vi "Copy Image To Picture.vi"(8 "error in (no error)":errorcluster, 10 "Transparency Threshold (127)":u8=127, 11 "image_ptr":i64) -> (0 "error out":errorcluster, 3 "Picture":T1)   [LabVIEW 2020, in "G-Image.lvlib"]
doc: "Read the image data from the pointer into LabVIEW, then free the memory. The image is returned as a LabVIEW picture."
uses:
  G-Image.lvlib
  <vilib>/picture/picture.llb/imagedata.ctl
  <vilib>/Utility/file.llb/Application Directory.vi
  <vilib>/Utility/error.llb/Error Cluster From Error Code.vi
  lib/g_image_32.dll
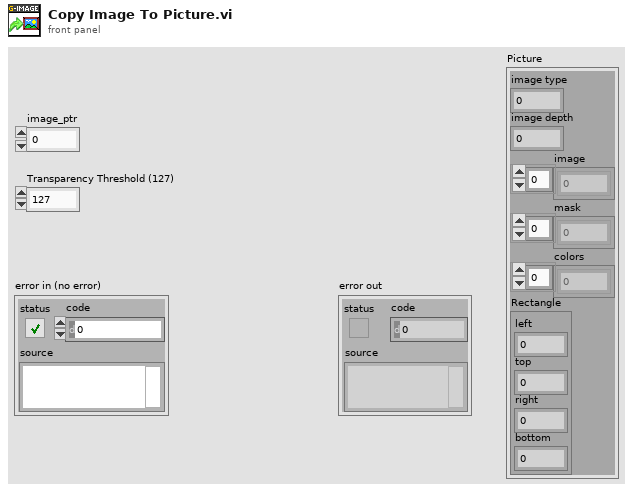
[diagram p1: front panel]
types:
  T1 = typedef "imagedata.ctl" = cluster{"image type":i32, "image depth":i32, "image":u8[], "mask":u8[], "colors":u32[], "Rectangle":cluster{"left":i16, "top":i16, "right":i16, "bottom":i16}}
  T2 = cluster{"data":i32, "colors":i32, "data_size":i32, "color_size":i32, "width":i32, "height":i32, "depth":i32}
  T3 = cluster{"data":i64, "colors":i64, "data_size":i32, "color_size":i32, "width":i32, "height":i32, "depth":i32}
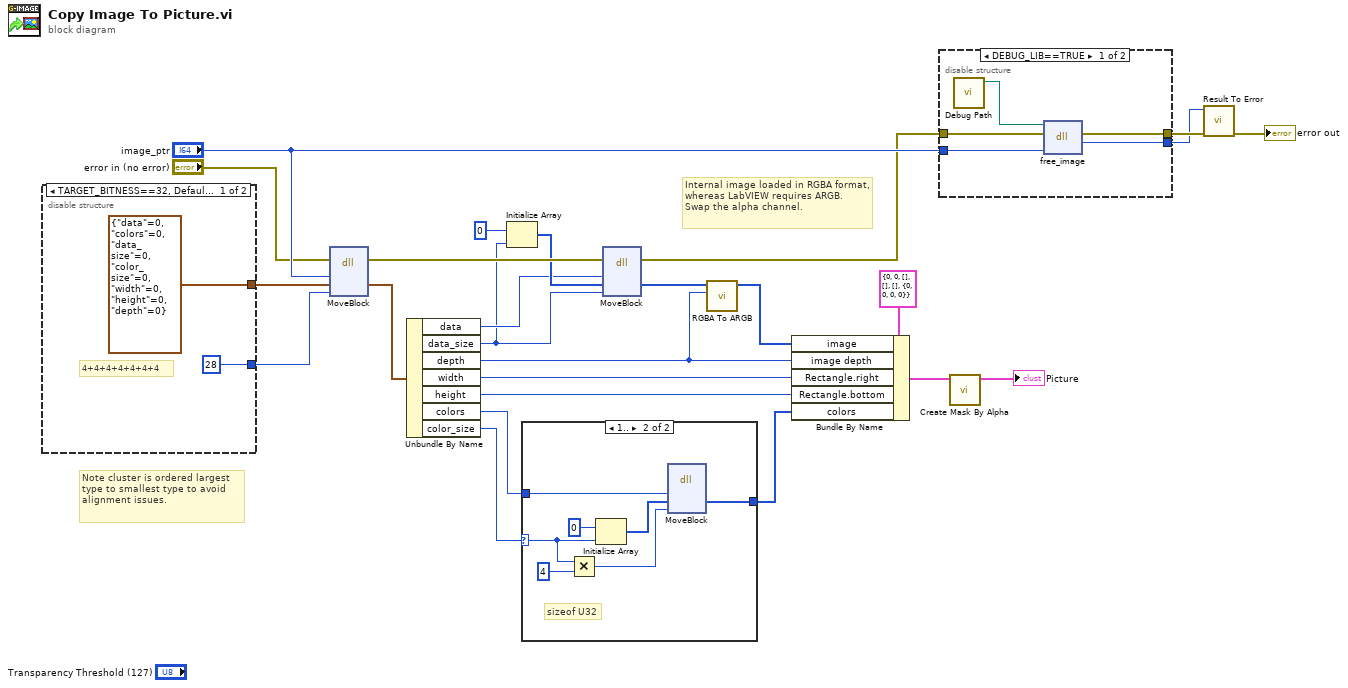
[diagram p0: block diagram]
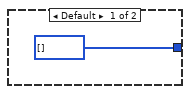
[diagram p2: hidden frame]
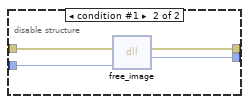
[diagram p3: hidden frame]
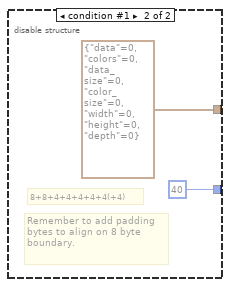
[diagram p4: hidden frame]
diagram:
  # "Internal image loaded in RGBA format, whereas LabVIEW requires ARGB. Swap the alpha channel."
  # "Note cluster is ordered largest type to smallest type to avoid alignment issues."
  n1 = disable-structure shown="TARGET_BITNESS==32, Default" {
    disable-tunnel: [T2 {"data"=0, "colors"=0, "data_size"=0, "color_size"=0, "width"=0, "height"=0, "depth"=0} T3 {"data"=0, "colors"=0, "data_size"=0, "color_size"=0, "width"=0, "height"=0, "depth"=0}] -> w17
    disable-tunnel: [28 ("x") 40 ("x")] -> w20
    frame condition #0 (active) {
      # "4+4+4+4+4+4+4"
    }
    frame condition #1 {
      # "Remember to add padding bytes to align on 8 byte boundary."
      # "8+8+4+4+4+4+4(+4)"
    }
  }
  n2 = dll-call lib="LabVIEW" fn="MoveBlock"(error in="error in (no error)", "Address (Pointer)"="image_ptr", "Destination"=w17, "Size"=w20) -> (error out=w21:errorcluster, "Destination"=w19:T2)  [unwired: 5 in, 1 out]
  n3 = Unbundle By Name(w19) -> ("data"=w14:i32, "data_size"=w11:i32, "depth"=w8:i32, "width"=w13:i32, "height"=w12:i32, "colors"=w4:i32, "color_size"=w3:i32)
  n4 = Initialize Array(u8 0 ("element"), w11) -> (w15:u8[])
  n5 = case shown="1.." w3 {
    selector: w3 -> [_ w31]
    tunnel: [u32[] [] ("Destination") w35] -> w5
    tunnel: w4 -> [_ w32]
    frame Default {
    }
    frame 1.. {
      # "sizeof U32"
      n6 = Multiply(x=w31, y=4) -> (x*y=w33:i32)
      n7 = Initialize Array(u32 0 ("element"), w31) -> (w37:u32[])
      n8 = dll-call lib="LabVIEW" fn="MoveBlock"("Address (Pointer)"=w32, "Destination"=w37, "Size"=w33) -> ("Destination"=w35:u32[])  [unwired: 6 in, 2 out]
    }
  }
  n9 = dll-call lib="LabVIEW" fn="MoveBlock"(error in=w21, "Address (Pointer)"=w14, "Destination"=w15, "Size"=w11) -> (error out=w18:errorcluster, "Destination"=w9:u8[])  [unwired: 5 in, 1 out]
  n10 = call "RGBA To ARGB.vi"("Depth"=w8, "RGBA"=w9) -> ("ARGB"=w7:u8[])  [unwired: 9 in]
  n11 = Bundle By Name(cluster=T1 {"image type"=0, "image depth"=0, "image"=[], "mask"=[], "colors"=[], "Rectangle"={"left"=0, "top"=0, "right"=0, "bottom"=0}} ("Pixmap"), "image"=w7, "image depth"=w8, "Rectangle.right"=w13, "Rectangle.bottom"=w12, "colors"=w5) -> (w2:T1)
  n12 = disable-structure shown="DEBUG_LIB==TRUE" {
    disable-tunnel: w18 -> [w41 w46]
    disable-tunnel: [w40 w45] -> w23
    disable-tunnel: [w39 w44] -> w22
    disable-tunnel: "image_ptr" -> [w38 w43]
    frame condition #0 (active) {
      n13 = call "Debug Path.vi"() -> ("Debug Path"=w42:path)  [unwired: 11 in]
      n14 = dll-call lib="?" fn="free_image"(path in=w42, error in=w41, "image_ptr"=w38) -> (error out=w40:errorcluster, "result"=w39:i32)  [unwired: 2 in, 1 out]
    }
    frame condition #1 {
      n15 = dll-call lib="C:/github/dataflowg/g-image/src/LabVIEW/G-Image/lib/g_image_*.*" fn="free_image"(error in=w46, "image_ptr"=w43) -> (error out=w45:errorcluster, "result"=w44:i32)  [unwired: 3 in, 1 out]
    }
  }
  n16 = call <vilib>:"Create Mask By Alpha.vi"("image data"=w2) -> ("masked image data"=→"Picture":T1)  [unwired: 10 in]
  n17 = call "Result To Error.vi"("error in (no error)"=w23, "Result Code"=w22) -> ("error out"=→"error out":errorcluster)  [unwired: 9 in]
